vi "HasTemplate.vi"(8 "error in (no error)":errorcluster, 11 "OneOfTemplate in":refnum<class "nidaqmx_grpc_SetChanAttributeStringRequest_attribute_enum.lvclass">) -> (0 "error out":errorcluster, 2 "Has Data?":bool, 3 "OneOfTemplate out":refnum<class "nidaqmx_grpc_SetChanAttributeStringRequest_attribute_enum.lvclass">)   [LabVIEW 2021, in "nidaqmx_grpc_SetChanAttributeStringRequest_attribute_enum.lvclass"]
uses:
  nidaqmx_grpc_SetChanAttributeStringRequest_attribute_enum.lvclass
  nidaqmx_grpc_SetChanAttributeStringRequest_attribute_enum.lvclass/nidaqmx_grpc_SetChanAttributeStringRequest_attribute_enum.ctl
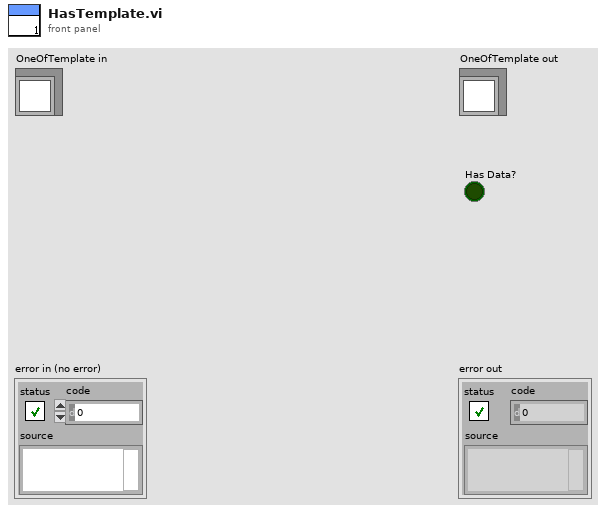
[diagram p1: front panel]
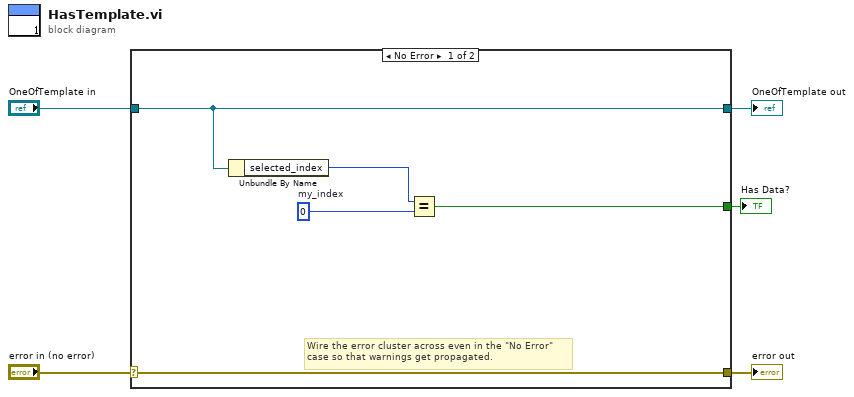
[diagram p0: block diagram]
diagram:
  n1 = case shown="No Error" "error in (no error)" {
    selector: "error in (no error)" -> [w10 w12]
    tunnel: [w10 w12] -> w4
    tunnel: [w9 w11] -> w2
    tunnel: "OneOfTemplate in" -> [w9 w11]
    tunnel: [w6 _] -> w1
    frame No Error {
      w7 = 0  # my_index
      # "Wire the error cluster across even in the \"No Error\"\ncase so that warnings get propagated."
      n2 = Unbundle By Name(w9) -> ("selected_index"=w8:i32)
      n3 = Equal?(x=w8, y=w7) -> (x = y?=w6:bool)
    }
    frame Error {
    }
  }
  "error out" <- w4
  "OneOfTemplate out" <- w2
  "Has Data?" <- w1
